vi "Celsius2Farenheit.vi"(0 "°C":dbl) -> (1 "stop 2":bool, 2 "°F":dbl)   [LabVIEW 2015]
panel:
  in  "stop":bool
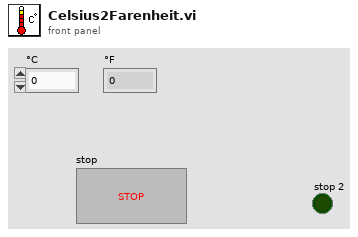
[diagram p1: front panel]
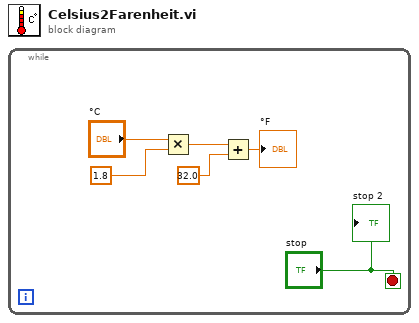
[diagram p0: block diagram]
diagram:
  n1 = while {
    stop <- "stop" stop-if-true
    n2 = Multiply(x="°C", y=1.8) -> (x*y=w5:dbl)
    n3 = Add(x=w5, y=32.0) -> (x+y=→"°F":dbl)
    "stop 2" <- "stop"
  }
